vi "Decay data normalizer.vi"(7 "avg wvfms":waveform(dbl)[](array[waveform])) -> (8 "norm avg wave":waveform(dbl))   [LabVIEW 2019]
doc: "This is a Bug C(T) subVI.\n\nThis subvi normalizes an exponential decay curve by subracting the baseline and then dividing by the first value, guaranteeing that the signal starts at 1.\n\nPaul K Dixon\nPhysics 3600\nCSUSB Physics"
uses:
  <vilib>/Analysis/baseanly.llb/Mean (DBL).vi
  <vilib>/Analysis/NI_AALBase.lvlib
panel:
  # "drive"
  # "Decay Normalizer"
  # "response"
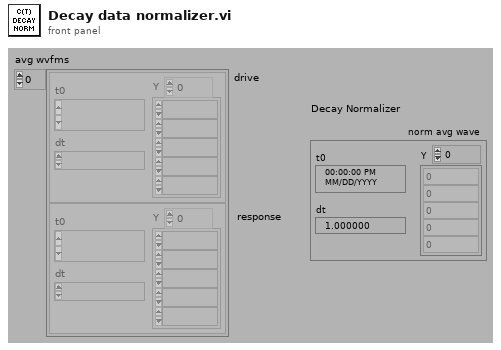
[diagram p1: front panel]
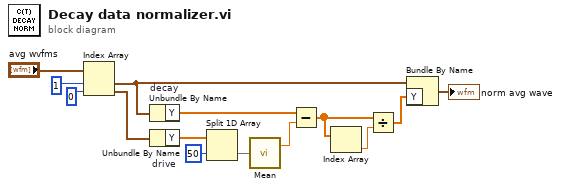
[diagram p0: block diagram]
diagram:
  n1 = Index Array(array="avg wvfms", index #1=1 ("Index (row)"), index #2=0 ("Index (row)")) -> (element #1=w2:waveform(dbl), element #2=w10:waveform(dbl))
  n2 = Unbundle By Name "decay"(w2) -> ("Y"=w7:dbl[])
  n3 = Unbundle By Name "drive"(w10) -> ("Y"=w9:dbl[])
  n4 = Split 1D Array(array=w9, index=50 ("Array Length")) -> (second subarray=w8:dbl[])  [unwired: 1 out]
  n5 = call-poly <vilib>:"Mean.vi"("X"=w8) -> ("mean"=w6:dbl)  [unwired: 1 out]
  n6 = Subtract(x=w7, y=w6) -> (x-y=w4:dbl[])
  n7 = Index Array(array=w4) -> (element=w5:dbl)  [unwired: 1 in]
  n8 = Divide(x=w4, y=w5) -> (x/y=w3:dbl[])
  n9 = Bundle By Name(cluster=w2, "Y"=w3) -> (→"norm avg wave":waveform(dbl))
